vi "initialise.vi"(8 "error in (no error)":errorcluster, 11 "GenericPlugin in":refnum<class "GenericImageAssembler.lvclass">) -> (0 "error out":errorcluster, 3 "GenericPlugin out":refnum<class "GenericImageAssembler.lvclass">)   [LabVIEW 2010, in "GenericImageAssembler.lvclass"]
doc: "The dynamic dispatch-version of this VI initalises the plug-in object by allocating and initalising any dynamic resources need."
uses:
  GenericImageAssembler.lvclass
  common/classes/GenericToplevelComponent/GenericToplevelComponent/GenericToplevelComponent.lvclass
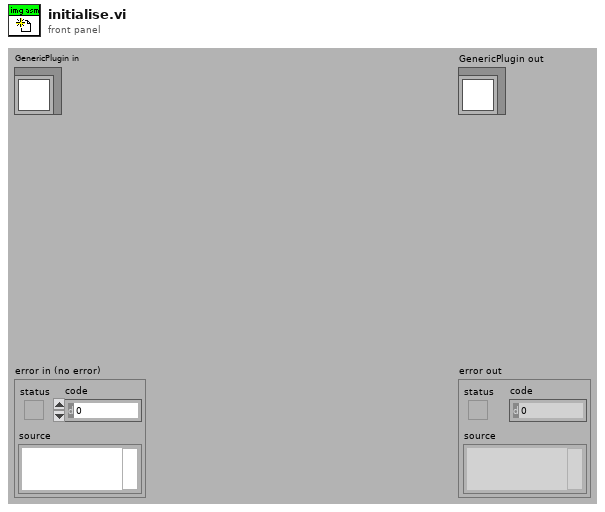
[diagram p1: front panel]
types:
  T1 = typedef "GenericToplevelComponent.lvclass/common_trigger_enum.ctl" = enum16{"NULL", "initialise", "terminate", "fetch command", "fetch data", "attach observer", "register as observer", "detach observer", "acknowledge", "start", "stop", "sweep started", "sweep finished", "experiment started", "experiment stopped"}
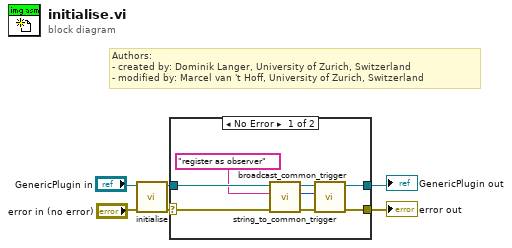
[diagram p0: block diagram]
diagram:
  # "Authors: \n- created by: Dominik Langer, University of Zurich, Switzerland\n- modified by: Marcel van 't Hoff, University of Zurich, Switzerland"
  n1 = call-parent "initialise.vi"("error in (no error)"="error in (no error)", "GenericPlugin in"="GenericPlugin in") -> ("error out"=w6:errorcluster, "GenericPlugin out"=w5:refnum<class "GenericImageAssembler.lvclass">)  [unwired: 8 in]
  n2 = case shown="No Error" w6 {
    selector: w6 -> [w9 w15]
    tunnel: w5 -> [w12 w16]
    tunnel: [w14 w15] -> w2
    tunnel: [w13 w16] -> w1
    frame No Error {
      n3 = call-dynamic "string_to_common_trigger.vi"("error in (no error)"=w9, "trigger string"="register as observer", "GenericToplevelComponent in"=w12) -> ("error out"=w8:errorcluster, "trigger"=w10:T1, "GenericToplevelComponent out"=w11:refnum<class "GenericImageAssembler.lvclass">)  [unwired: 6 in]
      n4 = call-dynamic "broadcast_common_trigger.vi"("error in (no error)"=w8, "trigger"=w10, "GenericToplevelComponent in"=w11) -> ("error out"=w14:errorcluster, "GenericToplevelComponent out"=w13:refnum<class "GenericImageAssembler.lvclass">)  [unwired: 7 in]
    }
    frame Error {
    }
  }
  "error out" <- w2
  "GenericPlugin out" <- w1
